vi "Initialize.vi"(8 "error in (no error)":errorcluster, 9 "Timeout [ms] (5000)":i32=5000, 10 "Connection":refnum<class "Connection.lvclass">, 11 "Connection in":refnum<class "Connection.lvclass">) -> (0 "error out":errorcluster, 3 "Connection out":refnum<class "Connection.lvclass">)   [LabVIEW 2022 SP3, in "Connection.lvlib" / "Connection.lvclass"]
uses:
  Connection.lvclass
  C:/Program Files (x86)/National Instruments/LabVIEW 2022/vi.lib/ActorFramework/Actor/Actor.lvclass
  C:/Users/jakub/repos/gh/sw4sys/lv-tcp-server-sample/LoggingActor/Source/LoggingActor/LoggingActor/LoggingActor.lvclass
  TcpSocket/Source/TcpSocket/Connection/Connection.lvclass
  Connection.lvclass/Connection.ctl
  _State.ctl
  <vilib>/ActorFramework/Actor/Actor.lvclass/Actor.ctl
  <vilib>/ActorFramework/Message Enqueuer/Message Enqueuer.lvclass/Message Enqueuer.ctl
  LoggingActor/Source/LoggingActor/LoggingActor/LoggingActor.lvclass/LoggingActor.ctl
  TcpSocket/Source/TcpSocket/Connection/Connection.lvclass/Connection.ctl
  TcpSocket/Source/TcpSocket/Connection/Read Address.vi
  TcpSocket/Source/TcpSocket/Connection/Read Port.vi
  TcpSocket/Source/TcpSocket/Connection/Read Connection.vi
  TcpSocket/Source/TcpSocket/Connection/Read ReadMode.vi
  TcpSocket/Source/TcpSocket/Connection/Read ReadTimeout.vi
  TcpSocket/Source/TcpSocket/Connection/Read WriteTimeout.vi
  LoggingActor/Source/LoggingActor/LoggingActor/Read Logger.vi
  <vilib>/ActorFramework/Message Enqueuer/Init from Existing Queue.vi
  <vilib>/ActorFramework/Message Enqueuer/Enqueue.vi
  Connection Messages/WaitForData Msg/WaitForData Msg.lvclass
  C:/Program Files (x86)/National Instruments/LabVIEW 2022/vi.lib/ActorFramework/Message/Message.lvclass
  <vilib>/ActorFramework/Message Priority Queue/Priority Enqueue.vi
  <vilib>/ActorFramework/Message Enqueuer/Message Enqueuer.lvclass
  Logger/Source/Logger/Logger.lvclass
  <vilib>/ActorFramework/Actor/Actor.lvclass
  C:/Users/jakub/repos/gh/sw4sys/lv-tcp-server-sample/TcpServerSample/Source/TcpServerSample/Connection/Connection/Connection.lvclass
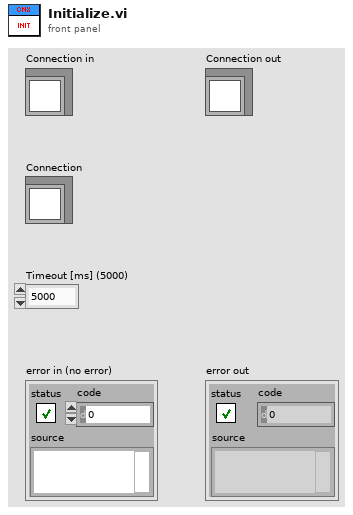
[diagram p1: front panel]
types:
  T1 = typedef "Connection.lvlib/Connection.lvclass/_State.ctl" = enum16{"WaitForInit", "Active", "Dying"}
  T2 = enum16{"Standard", "Buffered", "CRLF", "Immediate"}
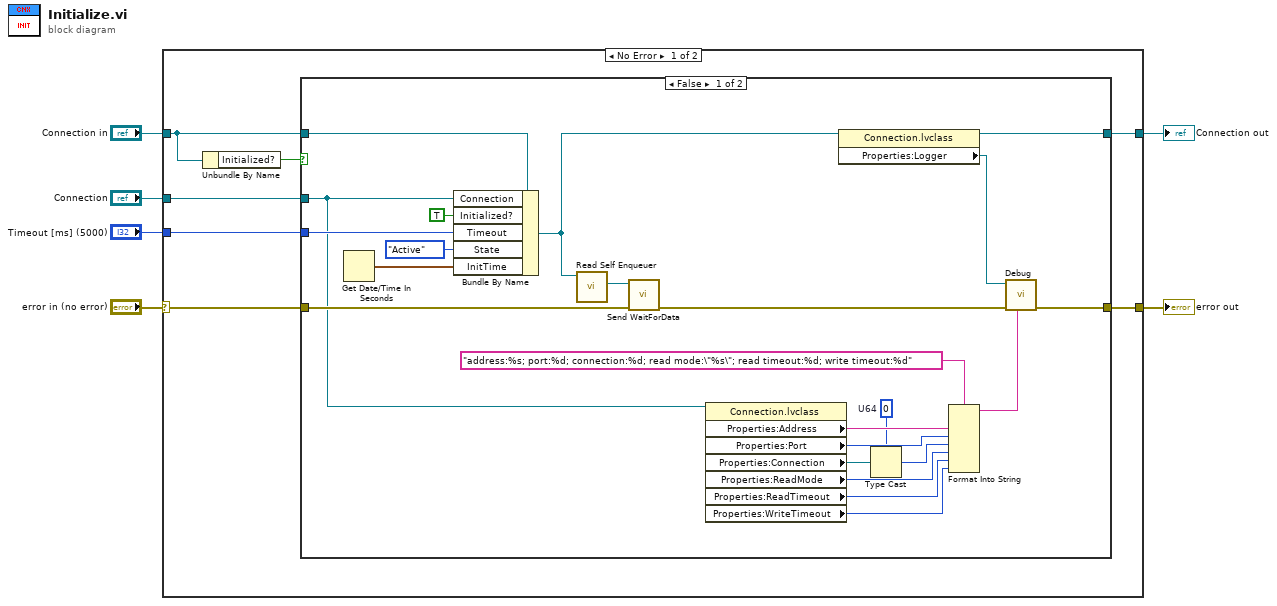
[diagram p0: block diagram]
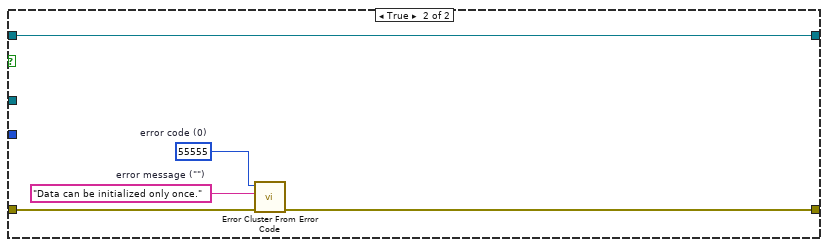
[diagram p2: hidden frame]
diagram:
  n1 = case shown="No Error" "error in (no error)" {
    selector: "error in (no error)" -> [w9 w43]
    tunnel: [w8 w43] -> w5
    tunnel: [w12 w42] -> w3
    tunnel: "Connection in" -> [w11 w42]
    tunnel: "Connection" -> [w13 _]
    tunnel: "Timeout [ms] (5000)" -> [w7 _]
    frame No Error {
      n2 = Unbundle By Name(w11) -> ("Initialized?"=w10:bool)
      n3 = case shown="False" w10 {
        tunnel: w13 -> [w24 _]
        tunnel: [w27 w41] -> w12
        tunnel: w11 -> [w35 w41]
        tunnel: w9 -> [w28 w40]
        tunnel: [w26 w39] -> w8
        tunnel: w7 -> [w34 _]
        frame False {
          w20 = u64 0  # U64
          n4 = Get Date/Time In Seconds() -> (seconds since 1Jan1904=w32:timestamp)
          n5 = Bundle By Name(cluster=w35, "Connection"=w24, "Initialized?"=TRUE, "Timeout"=w34, "State"=_State."Active", "InitTime"=w32) -> (w31:refnum<class "Connection.lvclass">)
          n6 = call <vilib>:"Read Self Enqueuer.vi"("Actor"=w31) -> ("Self Enqueuer"=w30:refnum<class "Message Enqueuer.lvclass">)  [unwired: 10 in]
          n7 = call "Send WaitForData.vi"("error in (no error)"=w28, "Message Enqueuer"=w30) -> ("error out"=w29:errorcluster)  [unwired: 8 in, 1 out]
          n8 = property class="Connection.lvclass"(reference=w24) -> ("Properties:Address"=w22:string, "Properties:Port"=w21:u16, "Properties:Connection"=w19:refnum<k5>, "Properties:ReadMode"=w17:T2, "Properties:ReadTimeout"=w16:i32, "Properties:WriteTimeout"=w15:i32)  [unwired: 1 in, 2 out]
          n9 = property class="Connection.lvclass"(reference=w31) -> (reference out=w27:refnum<class "Connection.lvclass">, "Properties:Logger"=w25:refnum<class "Logger.lvclass">)  [unwired: 1 in, 1 out]
          n10 = Type Cast(type=w20, x=w19) -> (*(type *) &x=w18:u64)
          n11 = Format Into String(format string="address:%s; port:%d; connection:%d; read mode:\"%s\"; read timeout:%d; write timeout:%d", w22, w21, w18, w17, w16, w15) -> (resulting string=w14:string)  [unwired: 2 in, 1 out]
          n12 = call-dynamic "Debug.vi"("Message"=w14, "error in (no error)"=w29, "Logger in"=w25) -> ("error out"=w26:errorcluster)  [unwired: 5 in, 1 out]
        }
        frame True {
          w37 = 55555  # error code (0)
          w38 = "Data can be initialized only once."  # error message ("")
          n13 = call <vilib>:"Error Cluster From Error Code.vi"("error in (no error)"=w40, "error message (\"\")"=w38, "error code (0)"=w37) -> ("error out"=w39:errorcluster)  [unwired: 6 in]
        }
      }
    }
    frame Error {
    }
  }
  "error out" <- w5
  "Connection out" <- w3
